vi "ADI_IMU_ADIS16448_AHRS_RoboBees.vi"(8 "Yaw Axis":enum16{"X", "Y", "Z"}(ring)=enum."Z", 9 "Delta t":dbl, 10 "Data 2":T2) -> (3 "Output":cluster{"Pitch":dbl, "Roll":dbl, "Yaw":dbl})   [LabVIEW 2019]
panel:
  out "Waveform Chart":T1(graph)
  in  "Tilt Comp (Yaw)":bool=TRUE
  in  "tau mag":dbl=0.04
  in  "tau acc":dbl=0.95
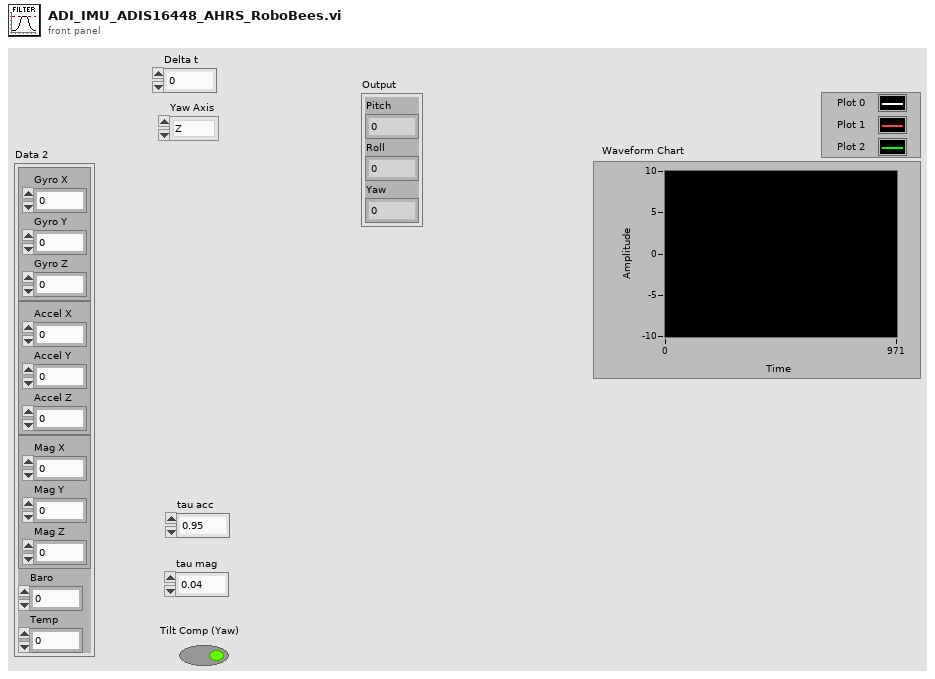
[diagram p1: front panel]
types:
  T1 = cluster{"XAngle":dbl, "YAngle":dbl, "ZAngle":dbl}
  T2 = cluster{cluster{"Gyro X":dbl, "Gyro Y":dbl, "Gyro Z":dbl}, cluster{"Accel X":dbl, "Accel Y":dbl, "Accel Z":dbl}, cluster{"Mag X":dbl, "Mag Y":dbl, "Mag Z":dbl}, "Baro":dbl, "Temp":dbl}
  T3 = cluster{"Xaccel":dbl, "Yaccel":dbl, "Zaccel":dbl}
  T4 = cluster{"Gyro X":dbl, "Gyro Y":dbl, "Gyro Z":dbl}
  T5 = cluster{"Accel X":dbl, "Accel Y":dbl, "Accel Z":dbl}
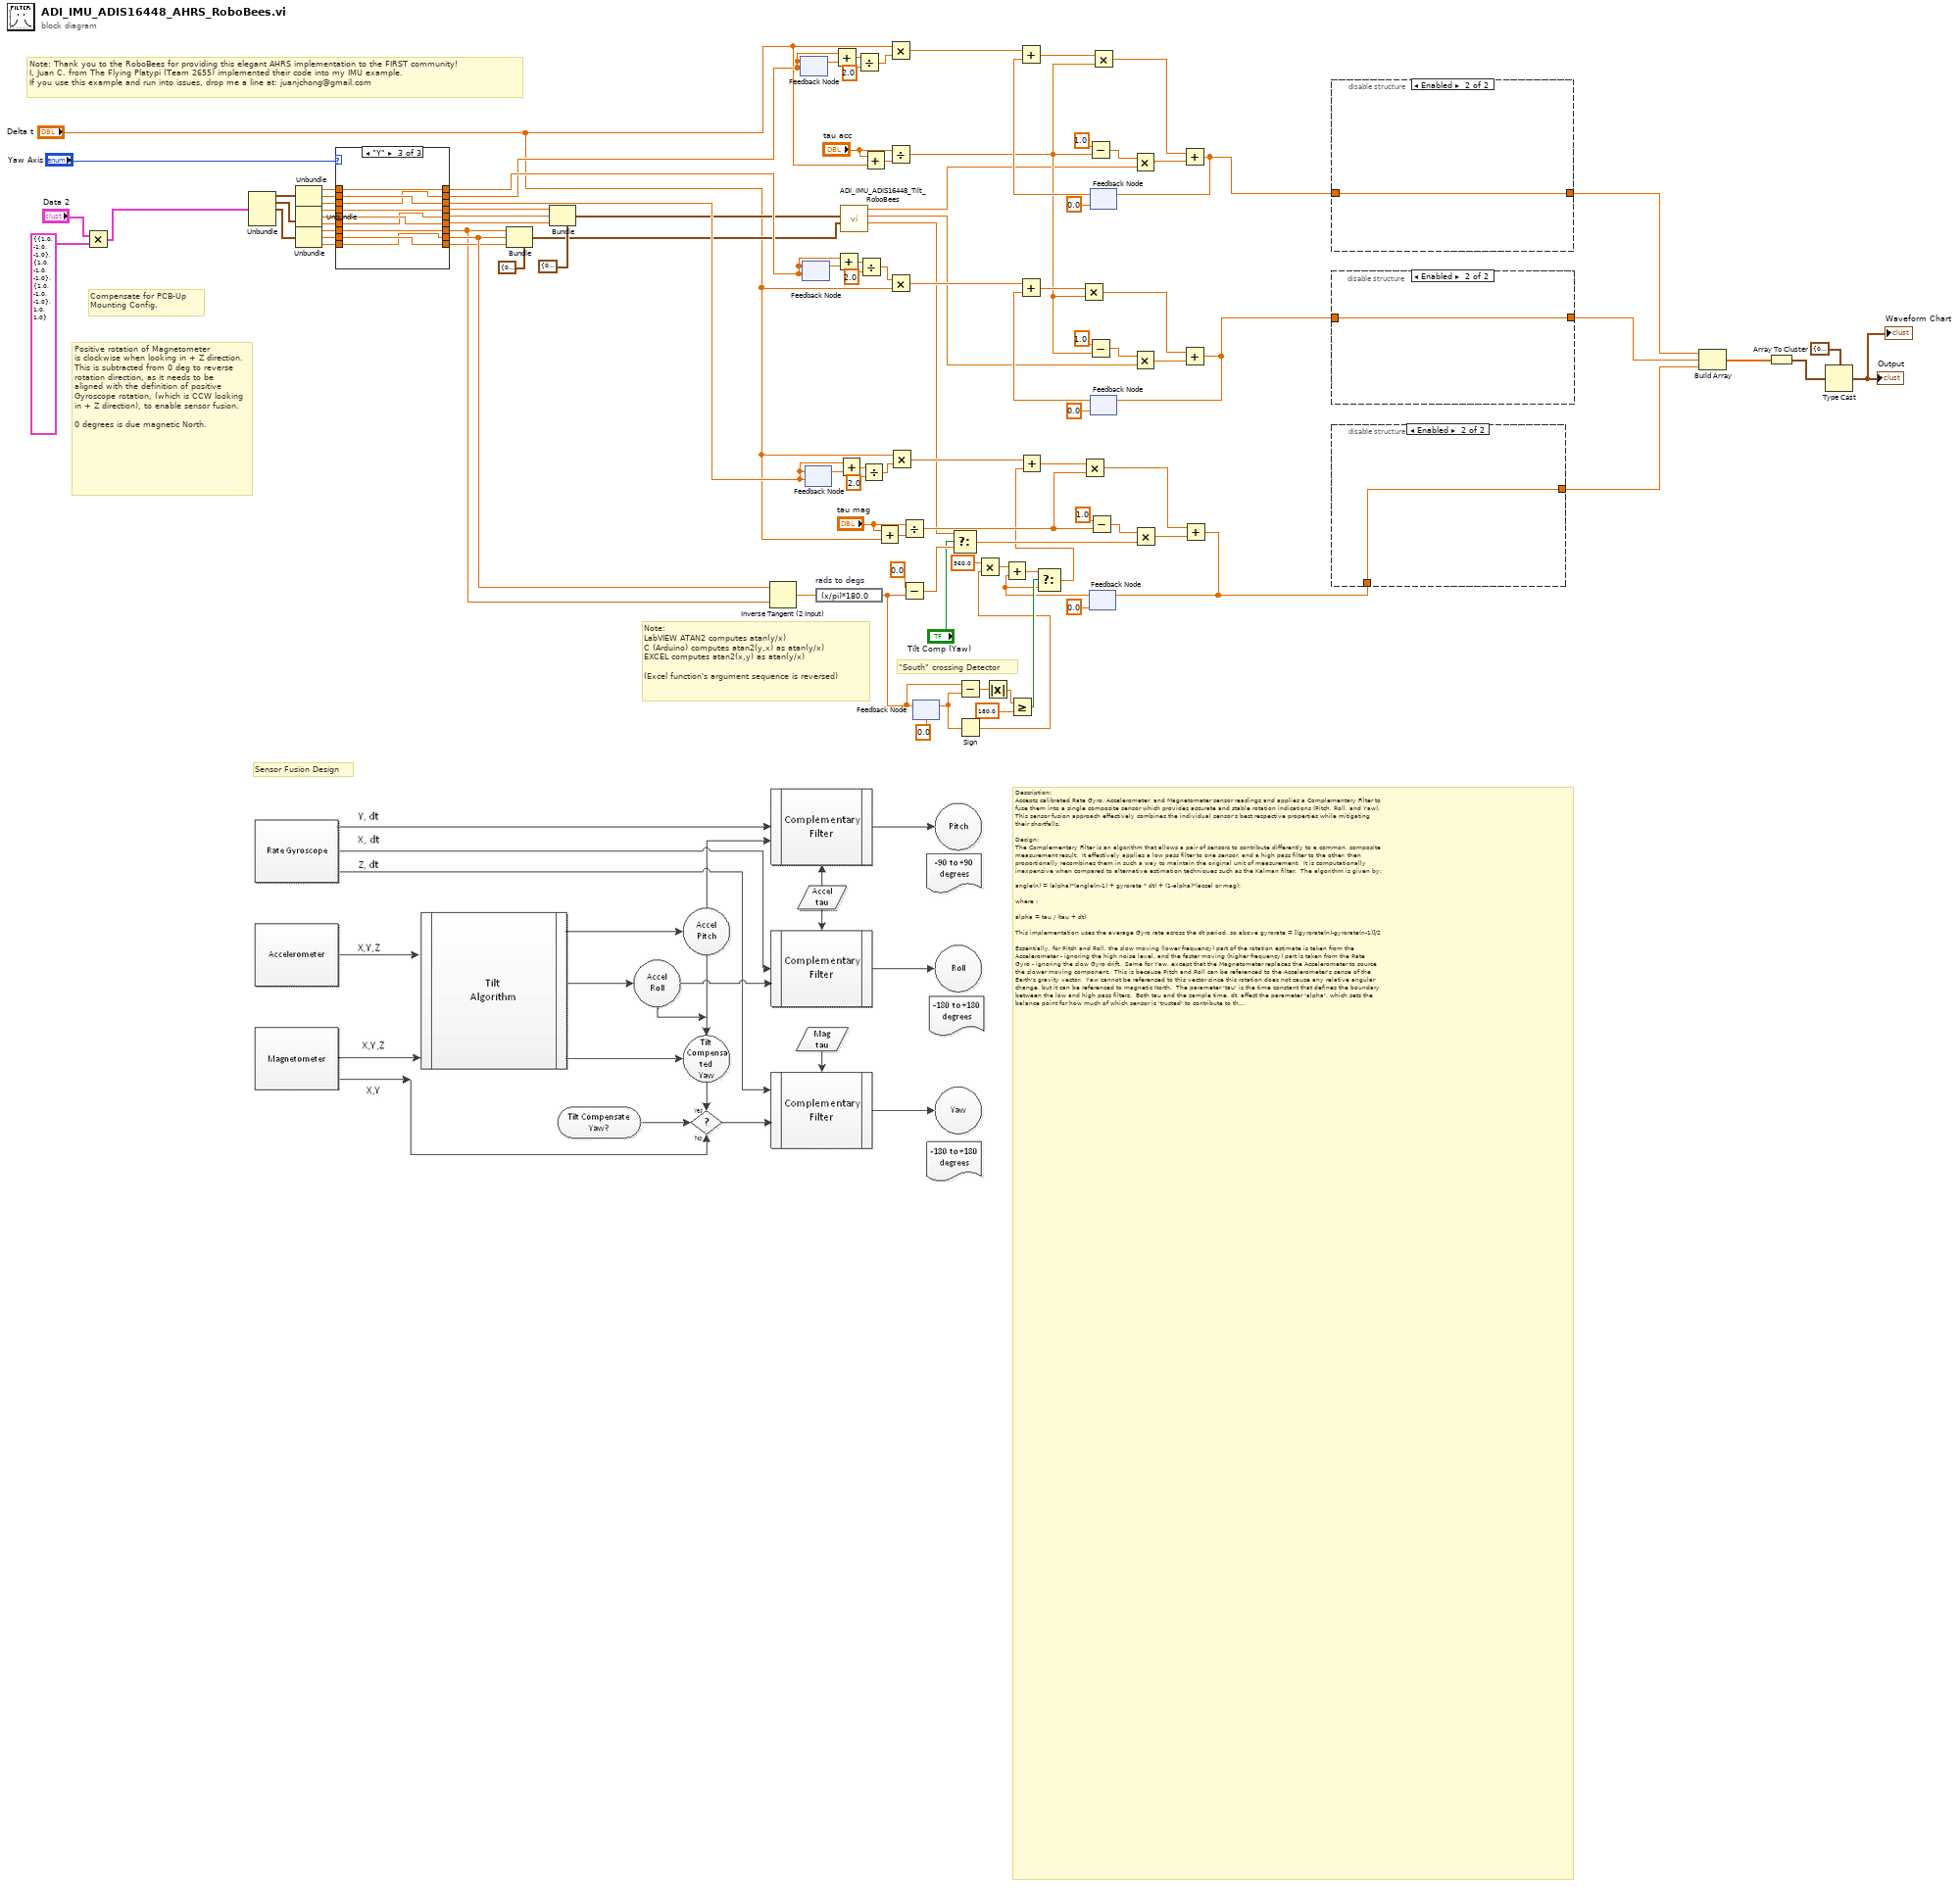
[diagram p0: block diagram]
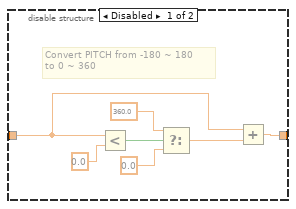
[diagram p2: hidden frame]
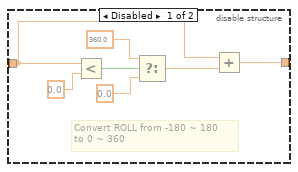
[diagram p3: hidden frame]
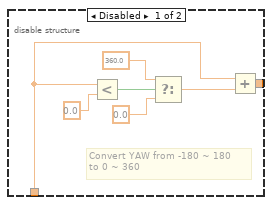
[diagram p4: hidden frame]
diagram:
  # "Compensate for PCB-Up\nMounting Config."
  # "Note: Thank you to the RoboBees for providing this elegant AHRS implementation to the FIRST community!\nI, Juan C. from The Flying Platypi (Team 2655) implemented their code into my IMU example.\nIf you use this example and run into issues, drop me a line at: juanjchong@gmail.com"
  # "Sensor Fusion Design"
  # "Description:\nAccepts calibrated Rate Gyro, Accelerometer, and Magnetometer sensor readings and applies a Complementary Filter to\nfuse them into a single composite sensor which provides accurate and stable rotation indications (Pitch, Roll, and Yaw).\nThis sensor fusion approach effectively combines the individual sensor's best respective properties while mitigating\ntheir shortfalls.\n\nDesign:\nThe Complementary Filter is an algorithm that allows a pair of sensors to contribute differently to a common, composite\nmeasurement result.  It effectively applies a low pass filter to one sensor, and a high pass filter to the other, then\nproportionally recombines them in such a way to maintain the original unit of measurement.  It is computationally\ninexpensive when compared to alternative estimation techniques such as the Kalman filter.  The algorithm is given by:\n\nangle(n) = (alpha)*(angle(n-1) + gyrorate * dt) + (1-alpha)*(accel or mag);\n\nwhere : \n\nalpha = tau / (tau + dt)\n\nThis implementation uses the average Gyro rate across the dt period, so above gyrorate = [(gyrorate(n)-gyrorate(n-1)]/2\n\nEssentially, for Pitch and Roll, the slow moving (lower frequency) part of the rotation estimate is taken from the\nAccelerometer - ignoring the high noise level, and the faster moving (higher frequency) part is taken from the Rate \nGyro - ignoring the slow Gyro drift.  Same for Yaw, except that the Magnetometer replaces the Accelerometer to source\nthe slower moving component.  This is because Pitch and Roll can be referenced to the Accelerometer's sense of the\nEarth's gravity vector.  Yaw cannot be referenced to this vector since this rotation does not cause any relative angular\nchange, but it can be referenced to magnetic North.  The parameter 'tau' is the time constant that defines the boundary\nbetween the low and high pass filters.  Both tau and the sample time, dt, affect the parameter 'alpha', which sets the\nbalance point for how much of which sensor is 'trusted' to contribute to the rotation estimate.\n\nThe Complementary Filter algorithm is applied to each X/Y/Z rotation axis to compute R/P/Y outputs, respectively.\n\nMagnetometer readings are tilt-compensated when Tilt-Comp-(Yaw) is asserted (True), by the IMU TILT subVI.  This\ncreates what is known as a tilt-compensated compass, which allows Yaw to be insensitive to the effects of a\nnon-level sensor, but generates error in Yaw during movement (coordinate acceleration).\n\nThe Yaw \"South\" crossing detector is necessary to allow a smooth transition across the +/- 180 deg discontinuity (inherent\nin the ATAN function).  Since -180 deg is congruent with +180 deg, Yaw needs to jump between these values when\ncrossing South (North is 0 deg).  The design depends upon comparison of successive Yaw readings to detect a cross-over\nevent.  The cross-over detector monitors the current reading and evaluates how far it is from the previous reading.  If it\nis greater than the previous reading by the Discriminant (= 180 deg), then Yaw just crossed South.\n\nBy choosing 180 as the Discriminant, the only way the detector can produce a false positive, assuming a loop iteration\nof 70 msec, is for it to rotate >2,571 dps ... (2,571=180/.07).  This is faster than the ST L3GD20 Gyro can register.  The\ndetector produces a Boolean True upon detecting a South crossing.  This is used to alter the (n-1) Yaw which was\npreviously stored, either adding or subtracting 360 degrees as required to place the previous Yaw in the correct quadrant\nwhenever crossing occurs.  The Modulus function cannot be used here as the Complementary Filter algorithm has 'state'\n(needs to remember previous Yaw).\n \nWe are in effect stitching together two ends of a ruler for 'modular arithmetic' (clock math).\n\nInputs:\nGYRO - Gyro rate and sample time measurements.\nACCEL - Acceleration measurements.\nMAG - Magnetic measurements.\nTAU ACC - tau parameter used to set sensor balance between Accel and Gyro for Roll and Pitch.\nTAU MAG -  tau parameter used to set sensor balance between Mag and Gyro for Yaw.\nTILT COMP (Yaw) - Enables Yaw tilt-compensation if True.\n\nOutputs:\nROLL - Filtered Roll about sensor X-axis.\nPITCH - Filtered Pitch about sensor Y-axis.\nYAW - Filtered Yaw about sensor Z-axis.\n\nVI Properties:\nExecution Reentrancy is set to Non Reentrant Execution\n\nImplementation:\nIt's best to establish the optimum loop sample time first.  See IMU READ implementation notes for guidance.  Each\ntau parameter should then be adjusted to achieve optimum sensor fusion.  tau acc affects Roll and Pitch, tau mag affects\nYaw.  Start at value 1 or 2 and decrease by half each time until the result doesn't drift, but not so far that the result gets\nnoisy.  An optimum tau for this IMU is likely in the range of 1.0 to 0.01, for a loop sample time between 10 and 100 ms.\n\nNote that both sample timing (dt) and tau both affect the balance parameter, 'alpha'.  Adjusting either dt or tau will\nrequire the other to be readjusted to maintain a particular filter performance.\n\nIt is likely best to set Yaw tilt-compensation to off (False) if the Yaw value is to be used as feedback in a closed loop\ncontrol application.  The tradeoff is that Yaw will only be accurate while the robot is level.\n\nSince a Yaw of -180 degrees is congruent with +180 degrees (they represent the same direction), it is possible that the\nYaw output will oscillate between these two values when the sensor happens to be pointing due South, as sensor\nnoise causes slight variation.  You will need to account for this possibility if you are using the Yaw value for decision-\nmaking in code.\n\n----- The RoboBees FRC Team 836! -----  Complement your passion to solve problems with a STEM Education!"
  # "\"South\" crossing Detector"
  # "Positive rotation of Magnetometer\nis clockwise when looking in + Z direction.  This is subtracted from 0 deg to reverse rotation direction, as it needs to be aligned with the definition of positive Gyroscope rotation, (which is CCW looking in + Z direction), to enable sensor fusion.\n\n0 degrees is due magnetic North."
  # "Note:\nLabVIEW ATAN2 computes atan(y/x)\nC (Arduino) computes atan2(y,x) as atan(y/x)\nEXCEL computes atan2(x,y) as atan(y/x)\n\n(Excel function's argument sequence is reversed)"
  n1 = Multiply(x="Data 2", y=T2 {{"Gyro X"=1.0, "Gyro Y"=-1.0, "Gyro Z"=-1.0}, {"Accel X"=1.0, "Accel Y"=-1.0, "Accel Z"=-1.0}, {"Mag X"=1.0, "Mag Y"=-1.0, "Mag Z"=-1.0}, "Baro"=1.0, "Temp"=1.0} ("Data 2")) -> (x*y=w2:T2)
  n2 = Unbundle(w2) -> (w16:T4, w15:T5, w14:cluster{"Mag X":dbl, "Mag Y":dbl, "Mag Z":dbl})  [unwired: 2 out]
  n3 = Unbundle(w16) -> ("Gyro X"=w13:dbl, "Gyro Y"=w12:dbl, "Gyro Z"=w11:dbl)
  n4 = Unbundle(w15) -> ("Accel X"=w10:dbl, "Accel Y"=w9:dbl, "Accel Z"=w8:dbl)
  n5 = Unbundle(w14) -> ("Mag X"=w7:dbl, "Mag Y"=w6:dbl, "Mag Z"=w5:dbl)
  n6 = case shown="\"Y\"" "Yaw Axis" {
    tunnel: [w105 w120 w129] -> w42
    tunnel: [w108 w117 w126] -> w35
    tunnel: [w111 w114 w123] -> w37
    tunnel: [w107 w116 w124] -> w34
    tunnel: [w106 w115 w125] -> w33
    tunnel: [w104 w119 w127] -> w41
    tunnel: [w103 w118 w128] -> w40
    tunnel: [w110 w113 w121] -> w39
    tunnel: [w109 w112 w122] -> w38
    tunnel: w13 -> [w103 w120 w129]
    tunnel: w12 -> [w104 w119 w128]
    tunnel: w11 -> [w105 w118 w127]
    tunnel: w10 -> [w106 w117 w126]
    tunnel: w9 -> [w107 w116 w125]
    tunnel: w8 -> [w108 w115 w124]
    tunnel: w7 -> [w109 w114 w123]
    tunnel: w6 -> [w110 w113 w122]
    tunnel: w5 -> [w111 w112 w121]
    frame "X" {
    }
    frame "Z", Default {
    }
    frame "Y" {
    }
  }
  n7 = Bundle(cluster=cluster{"Xmag":dbl, "Ymag":dbl, "Zmag":dbl} {"Xmag"=0.0, "Ymag"=0.0, "Zmag"=0.0} ("Mag"), "Xmag"=w37, "Ymag"=w39, "Zmag"=w38) -> (w30:cluster{"Xmag":dbl, "Ymag":dbl, "Zmag":dbl})
  n8 = Bundle(cluster=T3 {"Xaccel"=0.0, "Yaccel"=0.0, "Zaccel"=0.0} ("Accel"), "Xaccel"=w35, "Yaccel"=w34, "Zaccel"=w33) -> (w31:T3)
  n9 = Inverse Tangent (2 Input)(1:w37, 2:w39) -> (0:w75:dbl)
  n10 = feedback #1(w41) -> (w64:dbl)
  n11 = feedback-in #1(w41) -> ()
  n12 = feedback #2(w42) -> (w58:dbl)
  n13 = feedback-in #2(w42) -> ()
  n14 = feedback #3(w40) -> (w56:dbl)
  n15 = feedback-in #3(w40) -> ()
  n16 = expression code="(x/pi)*180.0" "rads to degs"(w75) -> (w45:dbl)
  n17 = Add(x=w41, y=w64) -> (x+y=w63:dbl)
  n18 = Add(x=w42, y=w58) -> (x+y=w59:dbl)
  n19 = Add(x=w40, y=w56) -> (x+y=w55:dbl)
  n20 = call "ADI_IMU_ADIS16448_Tilt_RoboBees.vi"("Mag"=w30, "Accel"=w31) -> ("Yaw"=w27:dbl, "Roll"=w28:dbl, "Pitch"=w29:dbl)  [unwired: 6 in, 1 out]
  n21 = Divide(x=w63, y=2.0) -> (x/y=w61:dbl)
  n22 = Divide(x=w59, y=2.0) -> (x/y=w57:dbl)
  n23 = Divide(x=w55, y=2.0) -> (x/y=w53:dbl)
  n24 = Add(x="tau acc", y="Delta t") -> (x+y=w101:dbl)
  n25 = Add(x="tau mag", y="Delta t") -> (x+y=w76:dbl)
  n26 = Multiply(x="Delta t", y=w61) -> (x*y=w89:dbl)
  n27 = Divide(x="tau acc", y=w101) -> (x/y=w85:dbl)
  n28 = Multiply(x=w57, y="Delta t") -> (x*y=w99:dbl)
  n29 = Multiply(x="Delta t", y=w53) -> (x*y=w69:dbl)
  n30 = Divide(x="tau mag", y=w76) -> (x/y=w68:dbl)
  n31 = Subtract(x=0.0 ("y"), y=w45) -> (x-y=w72:dbl)
  n32 = feedback #4(0.0) -> (w46:dbl)
  n33 = feedback-in #4(w45) -> ()
  n34 = Select(t=w27, s="Tilt Comp (Yaw)", f=w72) -> (s? t:f=w73:dbl)
  n35 = Subtract(x=w45, y=w46) -> (x-y=w52:dbl)
  n36 = Sign(1:w46) -> (0:w48:dbl)
  n37 = Multiply(x=360.0 ("y"), y=w48) -> (x*y=w44:dbl)
  n38 = Absolute Value(x=w52) -> (abs(x)=w51:dbl)
  n39 = Greater Or Equal?(x=w51, y=180.0) -> (x >= y?=w49:bool)
  n40 = Subtract(x=1.0, y=w85) -> (x-y=w88:dbl)
  n41 = Subtract(x=1.0, y=w85) -> (x-y=w84:dbl)
  n42 = Subtract(x=1.0, y=w68) -> (x-y=w82:dbl)
  n43 = feedback #5(0.0) -> (w43:dbl)
  n44 = Add(x=w44, y=w43) -> (x+y=w65:dbl)
  n45 = Select(t=w65, s=w49, f=w43) -> (s? t:f=w66:dbl)
  n46 = Add(x=w69, y=w66) -> (x+y=w79:dbl)
  n47 = Multiply(x=w79, y=w68) -> (x*y=w81:dbl)
  n48 = feedback #6(0.0) -> (w93:dbl)
  n49 = Add(x=w89, y=w93) -> (x+y=w90:dbl)
  n50 = Multiply(x=w90, y=w85) -> (x*y=w92:dbl)
  n51 = feedback #7(0.0) -> (w83:dbl)
  n52 = Add(x=w99, y=w83) -> (x+y=w98:dbl)
  n53 = Multiply(x=w98, y=w85) -> (x*y=w96:dbl)
  n54 = Multiply(x=w88, y=w29) -> (x*y=w91:dbl)
  n55 = Multiply(x=w84, y=w28) -> (x*y=w97:dbl)
  n56 = Multiply(x=w82, y=w73) -> (x*y=w80:dbl)
  n57 = Add(x=w92, y=w91) -> (x+y=w19:dbl)
  n58 = feedback-in #6(w19) -> ()
  n59 = Add(x=w96, y=w97) -> (x+y=w18:dbl)
  n60 = feedback-in #7(w18) -> ()
  n61 = Add(x=w81, y=w80) -> (x+y=w26:dbl)
  n62 = feedback-in #5(w26) -> ()
  n63 = disable-structure shown="Enabled" {
    disable-tunnel: w18 -> [w131 w137]
    disable-tunnel: [w130 w137] -> w24
    frame Disabled {
      # "Convert ROLL from -180 ~ 180 \nto 0 ~ 360"
      n64 = Less?(x=w131, y=0.0) -> (x < y?=w135:bool)
      n65 = Select(t=360.0, s=w135, f=0.0) -> (s? t:f=w132:dbl)
      n66 = Add(x=w131, y=w132) -> (x+y=w130:dbl)
    }
    frame Enabled {
    }
  }
  n67 = disable-structure shown="Enabled" {
    disable-tunnel: [w139 w145] -> w23
    disable-tunnel: w19 -> [w138 w145]
    frame Disabled {
      # "Convert PITCH from -180 ~ 180 \nto 0 ~ 360"
      n68 = Less?(x=w138, y=0.0) -> (x < y?=w143:bool)
      n69 = Select(t=360.0, s=w143, f=0.0) -> (s? t:f=w140:dbl)
      n70 = Add(x=w138, y=w140) -> (x+y=w139:dbl)
    }
    frame Enabled {
    }
  }
  n71 = disable-structure shown="Enabled" {
    disable-tunnel: w26 -> [w147 w153]
    disable-tunnel: [w146 w153] -> w25
    frame Disabled {
      # "Convert YAW from -180 ~ 180 \nto 0 ~ 360"
      n72 = Less?(x=w147, y=0.0) -> (x < y?=w151:bool)
      n73 = Select(t=360.0, s=w151, f=0.0) -> (s? t:f=w148:dbl)
      n74 = Add(x=w147, y=w148) -> (x+y=w146:dbl)
    }
    frame Enabled {
    }
  }
  n75 = Build Array(w23, w24, w25) -> (w20:dbl[])
  n76 = Array To Cluster(array=w20) -> (cluster=w21:cluster{"[0]":dbl, "[1]":dbl, "[2]":dbl})
  n77 = Type Cast(type=cluster{"Pitch":dbl, "Roll":dbl, "Yaw":dbl} {"Pitch"=0.0, "Roll"=0.0, "Yaw"=0.0} ("IMU AHRS"), x=w21) -> (*(type *) &x=→"Output" →"Waveform Chart":cluster{"Pitch":dbl, "Roll":dbl, "Yaw":dbl})
